vi "GetChannelplugged.vi"(8 "error in (no error)":errorcluster, 11 "ID In":i32) -> (0 "error out":errorcluster, 1 "FirstPluggedChannel":u8, 2 "PluggedChannels":u8[](array[numeric]), 3 "ID Out":i32, 4 "DisabledChannels":i32[](array[numeric]))   [LabVIEW 2022 SP3, in "EClib functions.lvlib"]
doc: "This VI returns the plugged channels."
uses:
  EClib functions.lvlib
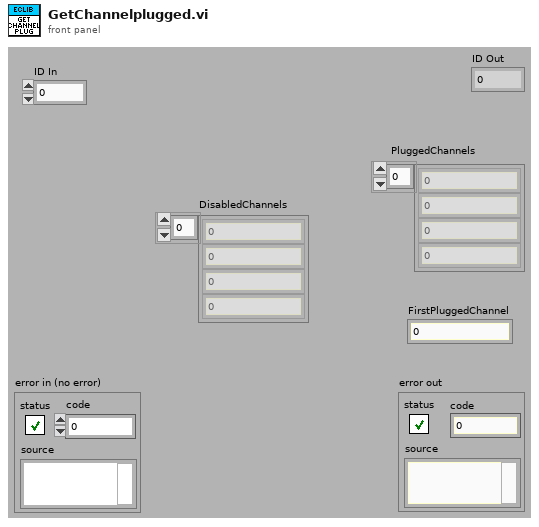
[diagram p1: front panel]
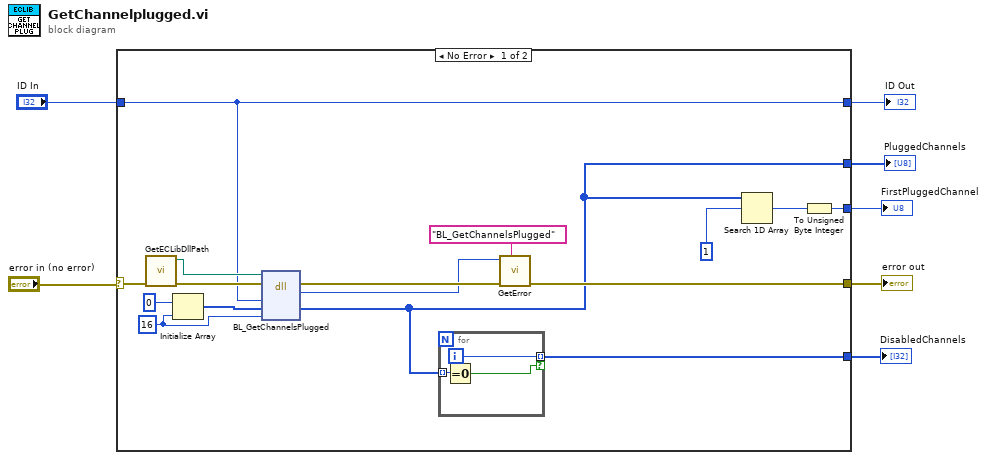
[diagram p0: block diagram]
diagram:
  n1 = case shown="No Error" "error in (no error)" {
    selector: "error in (no error)" -> [w14 w28]
    tunnel: [w18 w28] -> w6
    tunnel: "ID In" -> [w9 w27]
    tunnel: [w11 _] -> w4
    tunnel: [w8 _] -> w3
    tunnel: [w10 _] -> w2
    tunnel: [w9 w27] -> w1
    frame No Error {
      w22 = 16 ("dimension size")
      n2 = call "GetECLibDllPath.vi"("error in (no error)"=w14) -> ("error out"=w13:errorcluster, "ECLibDLLPath"=w19:path)  [unwired: 9 in]
      n3 = Initialize Array(0 ("element"), w22) -> (w20:i32[])
      n4 = dll-call lib="?" fn="BL_GetChannelsPlugged"(path in=w19, error in=w13, "arg1"=w9, "arg2"=w20, "arg3"=w22) -> (error out=w17:errorcluster, "return type"=w15:i32, "arg2"=w11:u8[])  [unwired: 3 in, 1 out]
      n5 = for {
        tunnel: w11 -> [w26] mode=indexing
        tunnel: [w25] -> w10 mode=indexing if=w24
        i -> [w25]
        n6 = Equal To 0?(x=w26) -> (x = 0?=w24:bool)
      }
      n7 = call "GetError.vi"("DLLFunction"="BL_GetChannelsPlugged", "error in"=w17, "code"=w15) -> ("error out"=w18:errorcluster)  [unwired: 8 in]
      n8 = Search 1D Array(1D array=w11, element=u8 1) -> (index of element=w12:i32)  [unwired: 1 in]
      n9 = To Unsigned Byte Integer(number=w12) -> (unsigned 8bit integer=w8:u8)
    }
    frame Error {
    }
  }
  "error out" <- w6
  "PluggedChannels" <- w4
  "FirstPluggedChannel" <- w3
  "DisabledChannels" <- w2
  "ID Out" <- w1
